vi "send command 01.vi"(8 "error in (no error)":errorcluster, 10 "command":string, 11 "IP address in":string="172.16.6.101") -> (0 "error out":errorcluster, 2 "response":string, 3 "IP address out":string="172.16.6.101")   [LabVIEW 2017]
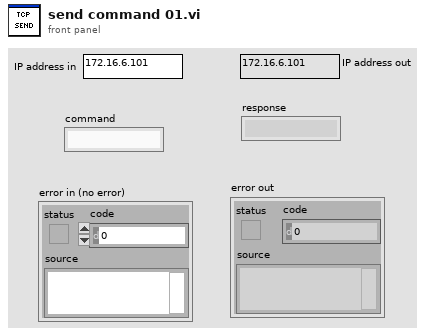
[diagram p1: front panel]
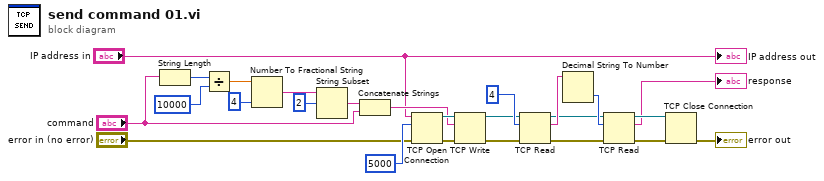
[diagram p0: block diagram]
diagram:
  n1 = String Length(string="command") -> (length=w22:i32)
  n2 = Divide(x=w22, y=10000) -> (x/y=w18:dbl)
  n3 = Number To Fractional String(number=w18, precision (6)=i16 4 ("Genauigkeit (6)")) -> (F-format string=w17:string)  [unwired: 2 in]
  n4 = String Subset(string=w17, offset (0)=2 ("Offset (0)")) -> (substring=w19:string)  [unwired: 1 in]
  n5 = Concatenate Strings(w19, "command") -> (w23:string)
  n6 = TCP Open Connection(address="IP address in", remote port or service name=u16 5000 ("Netzwerk-Port oder -Dienst"), error in (no error)="error in (no error)") -> (connection ID=w24:refnum<k5>, error out=w8:errorcluster)  [unwired: 2 in]
  n7 = TCP Write(connection ID=w24, data in=w23, error in (no error)=w8) -> (connection ID out=w11:refnum<k5>, error out=w7:errorcluster)  [unwired: 1 in, 1 out]
  n8 = TCP Read(connection ID=w11, bytes to read=4 ("Zu lesende Bytes"), error in (no error)=w7) -> (connection ID out=w12:refnum<k5>, data out=w14:string, error out=w6:errorcluster)  [unwired: 2 in]
  n9 = Decimal String To Number(string=w14) -> (number=w13:i32)  [unwired: 2 in, 1 out]
  n10 = TCP Read(connection ID=w12, bytes to read=w13, error in (no error)=w6) -> (connection ID out=w10:refnum<k5>, data out=→"response":string, error out=w5:errorcluster)  [unwired: 2 in]
  n11 = TCP Close Connection(connection ID=w10, error in (no error)=w5) -> (error out=→"error out":errorcluster)  [unwired: 1 in, 1 out]
  "IP address out" <- "IP address in"
